vi "File.Copy File to Root Folder using relative path as part of new name.vi"(8 "error in (no error)":errorcluster, 10 "Relative Path":string, 11 "Root Path":path) -> (0 "error out":errorcluster, 1 "Renamed":bool, 2 "New File Name":string, 3 "Adjusted Path":path)   [LabVIEW 2024]
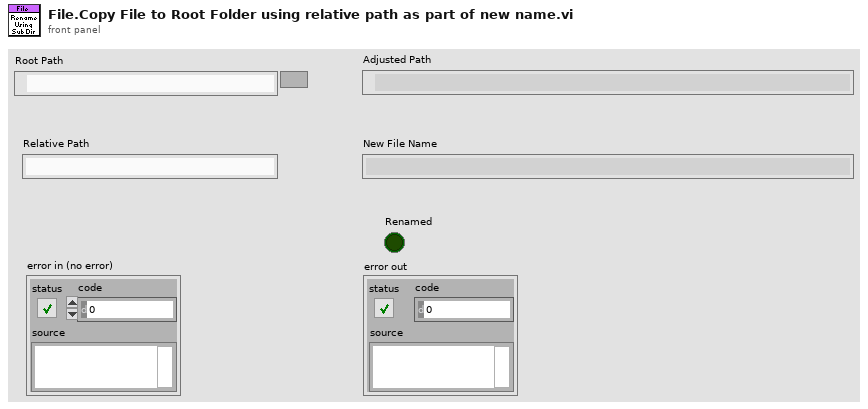
[diagram p1: front panel]
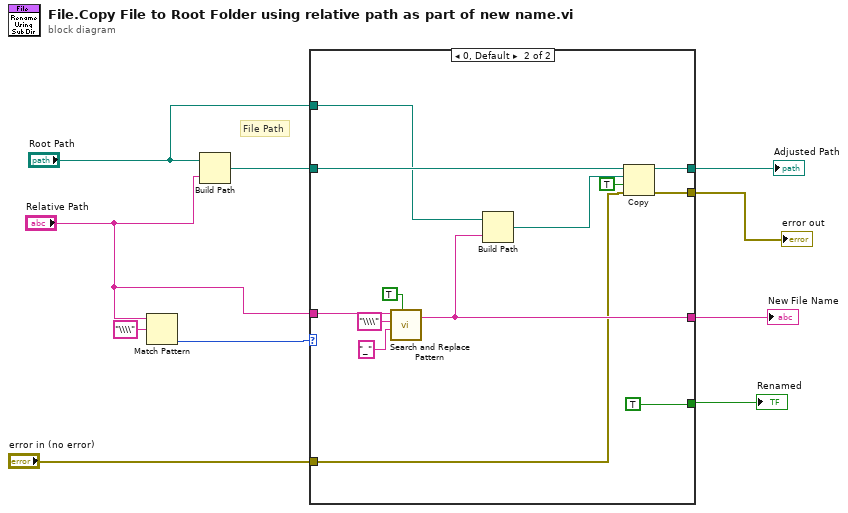
[diagram p0: block diagram]
diagram:
  # "File Path"
  n1 = Match Pattern(string="Relative Path", regular expression="\\\\") -> (offset past match=w4:i32)  [unwired: 1 in, 3 out]
  n2 = Build Path(base path="Root Path", name or relative path="Relative Path") -> (appended path=w8:path)
  n3 = case shown="0, Default" w4 {
    tunnel: "Relative Path" -> [w11 w24]
    tunnel: w8 -> [w12 w21]
    tunnel: [w12 w18] -> w7
    tunnel: [w11 w17] -> w6
    tunnel: "Root Path" -> [_ w16]
    tunnel: [_ TRUE] -> w3
    tunnel: [_ w14] -> w2
    tunnel: "error in (no error)" -> [_ w13]
    frame -1 {
    }
    frame 0, Default {
      n4 = call <vilib>:"Search and Replace Pattern.vi"("string"=w24, "regular expression (\"\")"="\\\\" ("regular expression (\"\")"), "replace string (\"\")"="_" ("replace string (\"\")"), "replace all? (F)"=TRUE) -> ("result string"=w17:string)  [unwired: 1 in, 1 out]
      n5 = Build Path(base path=w16, name or relative path=w17) -> (appended path=w20:path)
      n6 = Copy(8:w13, 9:TRUE ("overwrite (F)"), 10:w20, 11:w21) -> (0:w14:errorcluster, 3:w18:path)  [unwired: 1 in, 1 out]
    }
  }
  "Adjusted Path" <- w7
  "New File Name" <- w6
  "Renamed" <- w3
  "error out" <- w2
